vi "MT Format Eye Diagram (complex).vi"(0 "waveform":T1={"t0"=0.0, "dt"=1.0, "Y"=[]} {"Y" format="%.3f"; "dt" format="%^.2e"; "t0" format="%.4f"}, 1 "eye diagram reference":refnum<vi>, 5 "symbol rate (Hz)":dbl=1.0 format="%.2f", 7 "eye length":i32=1, 9 "I/Q (I)":enum16{"I", "Q"}(ring), 11 "error in (no error)":errorcluster, 12 "autoscale":bool) -> (4 "eye diagram":cluster{"t0":dbl, "dt":dbl, "Y":dbl[]}[](array[cluster]) {"Y" format="%.2f"; "dt" format="%.2f"; "t0" format="%.2f"}, 15 "error out":errorcluster)   [LabVIEW 2020, in "niDMT.lvlib"]
doc: "Specifies a complex-valued waveform, divides it into segments, and displays those segments as plots on a waveform graph. This VI determines the segment length based on the <B>symbol rate</B> and <B>eye length</B> parameters."
uses:
  <vilib>/addons/Modulation/niDMT.lvlib
  <vilib>/addons/Modulation/Analog/controls/Complex Data Waveform.ctl
  <vilib>/addons/Modulation/Digital/General/subVIs/mod_Segment Array(real).vi
  <vilib>/addons/Modulation/niAMT.lvlib
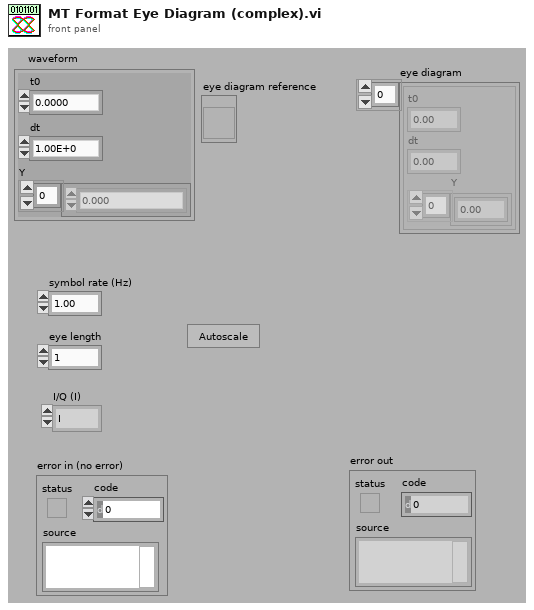
[diagram p1: front panel]
types:
  T1 = typedef "niAMT.lvlib/Complex Data Waveform.ctl" = cluster{"t0":dbl, "dt":dbl, "Y":cdb[]}
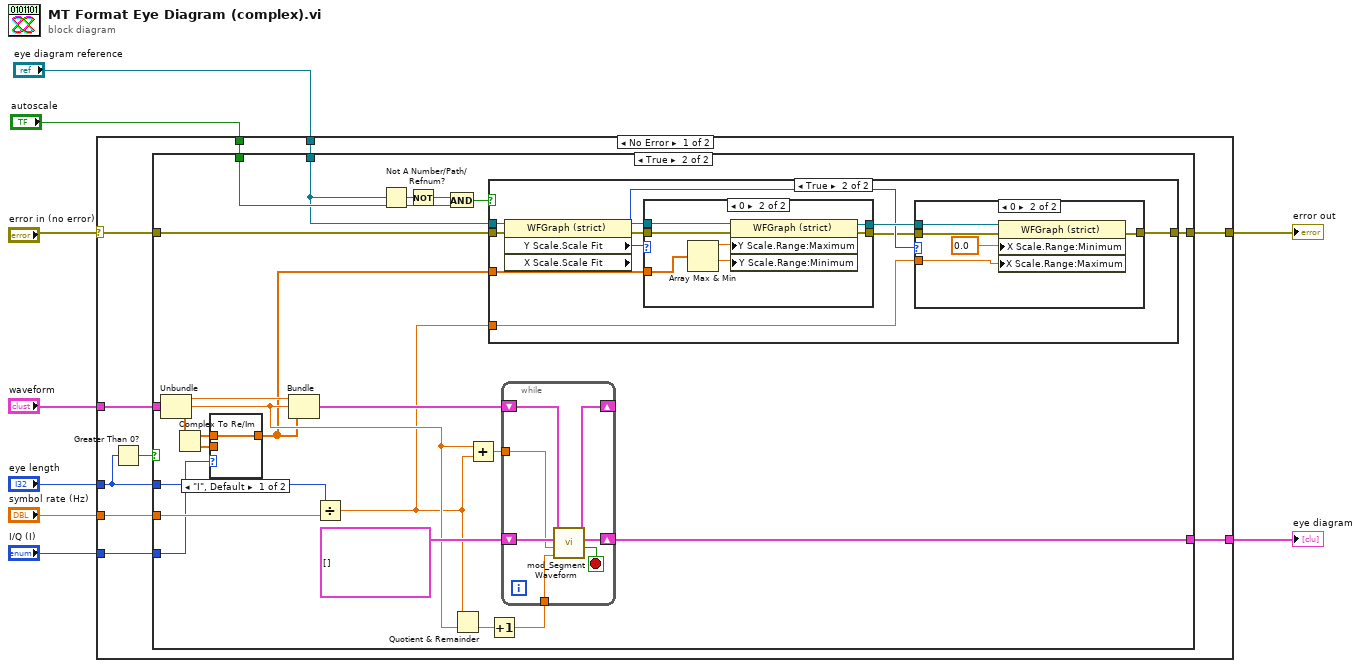
[diagram p0: block diagram]
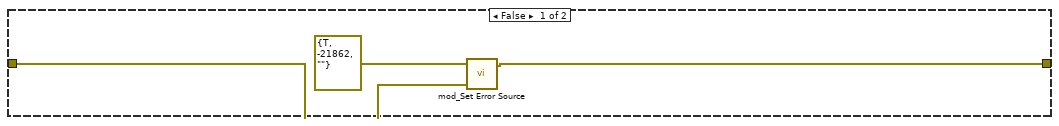
[diagram p2: hidden frame]
diagram:
  n1 = case shown="No Error" "error in (no error)" {
    selector: "error in (no error)" -> [w11 w83]
    tunnel: "eye length" -> [w13 _]
    tunnel: "symbol rate (Hz)" -> [w19 _]
    tunnel: [w18 _] -> w7
    tunnel: "waveform" -> [w17 _]
    tunnel: "I/Q (I)" -> [w14 _]
    tunnel: [w10 w83] -> w3
    tunnel: "autoscale" -> [w16 _]
    tunnel: "eye diagram reference" -> [w15 _]
    frame No Error {
      n2 = Greater Than 0?(x=w13) -> (x > 0?=w12:bool)
      n3 = case shown="True" w12 {
        tunnel: w19 -> [_ w46]
        tunnel: [_ w33] -> w18
        tunnel: w17 -> [_ w42]
        tunnel: w16 -> [_ w32]
        tunnel: w15 -> [_ w24]
        tunnel: w11 -> [w20 w23]
        tunnel: [w21 w28] -> w10
        tunnel: w14 -> [_ w35]
        tunnel: w13 -> [_ w34]
        frame False {
          n4 = call <vilib>:"mod_Set Error Source.vi"("initial error in (no error)"=w20, "final error in (no error)"=errorcluster {"status"=TRUE, "code"=-21862, "source"=""}) -> ("error out"=w21:errorcluster)  [unwired: 3 out]
        }
        frame True {
          n5 = Unbundle(w42) -> ("t0"=w41:dbl, "dt"=w38:dbl, "Y"=w40:cdb[])
          n6 = Complex To Re/Im(x + iy=w40) -> (x=w36:dbl[], y=w37:dbl[])
          n7 = case shown="\"I\", Default" w35 {
            tunnel: [w74 w75] -> w26
            tunnel: w36 -> [w74 _]
            tunnel: w37 -> [_ w75]
            frame "I", Default {
            }
            frame "Q" {
            }
          }
          n8 = Bundle("t0"=w41, "dt"=w38, w26) -> (w39:cluster{"t0":dbl, "dt":dbl, dbl[]})  [unwired: 1 out]
          n9 = Divide(x=w34, y=w46) -> (x/y=w27:dbl)
          n10 = Not A Number/Path/Refnum?(number/path/refnum=w24) -> (NaN/Path/Refnum?=w31:bool)
          n11 = Not(x=w31) -> (.not. x?=w30:bool)
          n12 = And(x=w30, y=w32) -> (x .and. y?=w25:bool)
          n13 = Quotient & Remainder(x=w27, y=w38) -> (floor(x/y)=w45:dbl)  [unwired: 1 out]
          n14 = Add(x=w38, y=w27) -> (x+y=w29:dbl)
          n15 = case shown="True" w25 {
            tunnel: [w47 w48] -> w28
            tunnel: w24 -> [_ w57]
            tunnel: w23 -> [w47 w56]
            tunnel: w26 -> [_ w58]
            tunnel: w27 -> [_ w50]
            frame False {
            }
            frame True {
              n16 = property class="WFGraph (strict)"(reference=w57, error in=w56) -> (reference out=w55:refnum<vi>, error out=w54:errorcluster, "Y Scale.Scale Fit"=w53:u8, "X Scale.Scale Fit"=w51:u8)
              n17 = case shown="0" w53 {
                tunnel: [w66 w73] -> w49
                tunnel: w58 -> [_ w72]
                tunnel: w55 -> [w65 w71]
                tunnel: w54 -> [w66 w70]
                tunnel: [w65 w69] -> w52
                frame 1, Default {
                }
                frame 0 {
                  n18 = Array Max & Min(array=w72) -> (max value=w68:dbl, min value=w67:dbl)  [unwired: 2 out]
                  n19 = property class="WFGraph (strict)"(reference=w71, error in=w70, "Y Scale.Range:Maximum"=w68, "Y Scale.Range:Minimum"=w67) -> (reference out=w69:refnum<vi>, error out=w73:errorcluster)
                }
              }
              n20 = case shown="0" w51 {
                tunnel: [w59 w60] -> w48
                tunnel: w50 -> [_ w63]
                tunnel: w52 -> [_ w62]
                tunnel: w49 -> [w59 w61]
                frame 1, Default {
                }
                frame 0 {
                  n21 = property class="WFGraph (strict)"(reference=w62, error in=w61, "X Scale.Range:Minimum"=0.0, "X Scale.Range:Maximum"=w63) -> (error out=w60:errorcluster)  [unwired: 1 out]
                }
              }
            }
          }
          n22 = Increment(x=w45) -> (x+1=w43:dbl)
          n23 = while {
            tunnel: w29 -> [w79]
            tunnel: w43 -> [w78]
            shift-right: [w81] -> _
            shift-left: w39 -> [w82]
            shift-right: [w76] -> w33
            shift-left: cluster{"t0":dbl, "dt":dbl, "Y":dbl[]}[] [] ("empty graphs in") -> [w80]
            stop <- w77 stop-if-true
            n24 = call-poly <vilib>:"mod_Segment Waveform.vi"("min samples per segment"=w78, "segment time"=w79, "graphs in"=w80, "waveform"=w82) -> ("done?"=w77:bool, "graphs out"=w76:cluster{dbl, "dt":dbl, dbl[]}[], "waveform out"=w81:cluster{"t0":dbl, "dt":dbl, "Y":dbl[]})  [unwired: 5 out]
          }
        }
      }
    }
    frame Error {
    }
  }
  "eye diagram" <- w7
  "error out" <- w3
